vi "Display Settings.vi"() -> ()   [LabVIEW 2013, in "Stanford Research CG635.lvlib"]
uses:
  <instrlib>/Stanford Research CG635/Stanford Research CG635.lvlib
panel:
  in  "Units":u16(ring) items=["Hz", "kHz", "MHz", "GHz"]
  in  "Display Value":u16(ring) items=["Frequency", "Phase", "Q /Q High", "Q / Q Low", "CMOS High", "CMOS Low", "Frequency Step", "Phase Step", "Q / Q High Step", "Q / Q Low Step", "CMOS High Step", "CMOS Low Step"]
  out "VISA resource name out":refnum<visa-resource-name>
  out "error out":errorcluster
  in  "VISA resource name":refnum<visa-resource-name>
  in  "error in (no error)":errorcluster
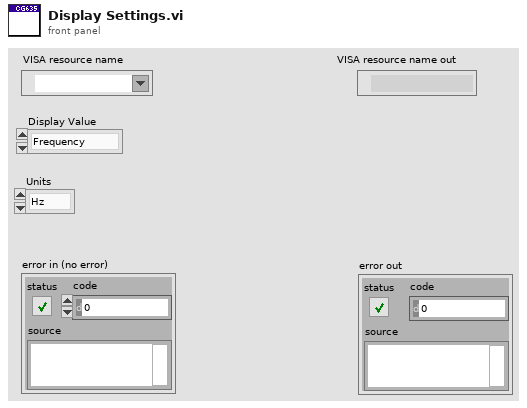
[diagram p1: front panel]
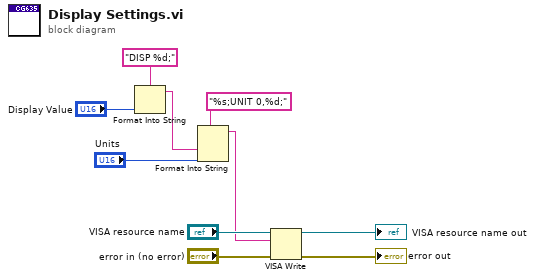
[diagram p0: block diagram]
diagram:
  n1 = Format Into String(format string="DISP %d;", "Display Value") -> (resulting string=w4:string)  [unwired: 2 in, 1 out]
  n2 = Format Into String(format string="%s;UNIT 0,%d;", w4, "Units") -> (resulting string=w1:string)  [unwired: 2 in, 1 out]
  n3 = VISA Write(VISA resource name="VISA resource name", write buffer=w1, error in (no error)="error in (no error)") -> (VISA resource name out=→"VISA resource name out":refnum<visa-resource-name>, error out=→"error out":errorcluster)  [unwired: 1 out]
